vi "Create Block Set Address (SubVI).vi"(0 "Image Width":u16, 5 "Block Size":u16, 8 "Block N":u16, 10 "Block Y":u16, 12 "Block X":u16) -> (14 "Address":u16)   [LabVIEW 2015]
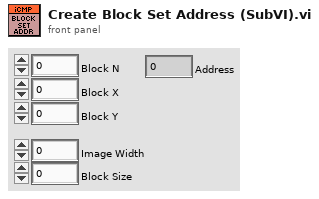
[diagram p1: front panel]
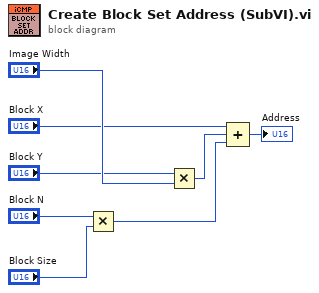
[diagram p0: block diagram]
diagram:
  n1 = Multiply(x="Block N", y="Block Size") -> (x*y=w6:u16)
  n2 = Multiply(x="Block Y", y="Image Width") -> (x*y=w5:u16)
  n3 = Compound Arithmetic op=ADD("Block X", w5, w6) -> (→"Address":u16)
